vi "Realtime_interaction VI.vi"() -> ()   [LabVIEW 2020]
uses:
  <vilib>/FPGAPlugInAG/cRIO-9054/niLvFpga_Open_cRIO-9054.vi
  <vilib>/rvi/interface/common/dynamic/niFpgaDynamicAddResources.vi
  <vilib>/Utility/error.llb/Error Cluster From Error Code.vi
  <vilib>/rvi/errors/niLvFpgaAdjustHostInterfaceError.vi
  <vilib>/FPGAPlugInAG/Dynamic/niLvFpga_Close_Dynamic.vi
  <vilib>/rvi/interface/nirviOpenFPGA/nirviOpenFPGA.xnode
  secondarytest track hostsytem at helios/FPGA Bitfiles/modifiedtestproj_FPGATarget_FPGAcontrolledVI_2pmID5UxXW8.lvbitx
  secondarytest track hostsytem at helios/FPGA_controlled VI.vi
  <vilib>/rvi/interface/nirviReadWriteControl/nirviReadWriteControl.xnode
  <vilib>/rvi/interface/nirviCloseFPGA/nirviCloseFPGA.xnode
  NiFpgaLv.dll
  <vilib>/rvi/interface/Simulation/niFpgaSimulationCallBeginRW.vi
panel:
  out "Numeric 2":fxp<+/-,20,5> format="%#_5f"
  in  "stop":bool
  in  "Horizontal Pointer Slide":dbl(slide) scale=0.0..10.0 scale format="%#2_3g"
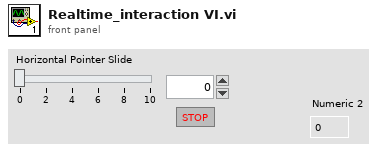
[diagram p1: front panel]
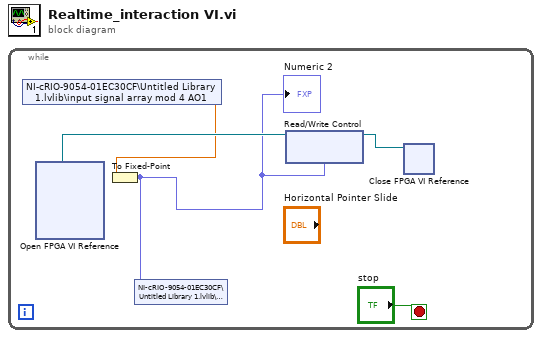
[diagram p0: block diagram]
diagram:
  n1 = while {
    stop <- "stop" stop-if-true
    n2 = shared-variable "NI-cRIO-9054-01EC30CF\\Untitled Library 1.lvlib\\input signal array mod 4 AO1"() -> (w2:dbl)  [unwired: 1 in, 1 out]
    n3 = xnode "Open FPGA VI Reference"() -> ("FPGA VI Reference Out"=w3:refnum<k20>)  [unwired: 2 in, 1 out]
    n4 = To Fixed-Point(number=w2) -> (fixed-point=w1:fxp<+/-,20,5>)  [unwired: 1 in]
    "Numeric 2" <- w1
    n5 = shared-variable "NI-cRIO-9054-01EC30CF\\Untitled Library 1.lvlib\\readback"(w1) -> ()  [unwired: 1 in, 1 out]
    n6 = xnode "Read/Write Control"("FPGA VI Reference In"=w3, "Mod4/AO0"=w1) -> ("FPGA VI Reference Out"=w4:refnum<k20>)  [unwired: 1 in, 1 out]
    n7 = xnode "Close FPGA VI Reference"("FPGA VI Reference In"=w4) -> ()  [unwired: 1 in, 1 out]
  }
